vi "Trapezoidal Acceleration.vi"(9 "Desired":dbl, 10 "Actual":dbl) -> (2 "New Actual":dbl)   [LabVIEW 2013]
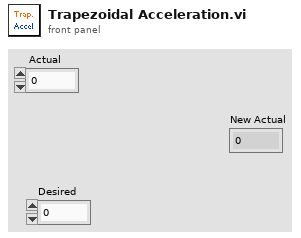
[diagram p1: front panel]
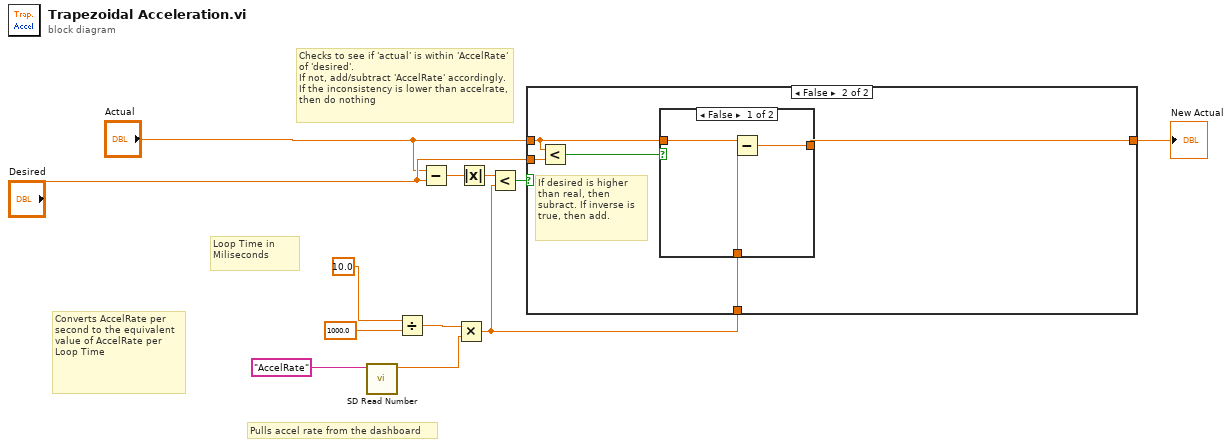
[diagram p0: block diagram]
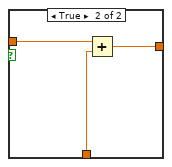
[diagram p3: hidden frame]
diagram:
  # "Pulls accel rate from the dashboard"
  # "Checks to see if 'actual' is within 'AccelRate' of 'desired'.\nIf not, add/subtract 'AccelRate' accordingly. If the inconsistency is lower than accelrate, then do nothing"
  # "Converts AccelRate per second to the equivalent value of AccelRate per Loop Time"
  # "Loop Time in Miliseconds"
  n1 = call <vilib>:"SD Read Number.vi"("Name"="AccelRate") -> ("Numeric"=w2:dbl)  [unwired: 8 in, 2 out]
  n2 = Divide(x=10.0, y=1000.0) -> (x/y=w8:dbl)
  n3 = Subtract(x="Actual", y="Desired") -> (x-y=w11:dbl)
  n4 = Multiply(x=w8, y=w2) -> (x*y=w6:dbl)
  n5 = Absolute Value(x=w11) -> (abs(x)=w12:dbl)
  n6 = Less?(x=w12, y=w6) -> (x < y?=w10:bool)
  n7 = case shown="False" w10 {
    tunnel: [w13 w18] -> w5
    tunnel: "Actual" -> [w13 w17]
    tunnel: "Desired" -> [_ w15]
    tunnel: w6 -> [_ w14]
    frame True {
    }
    frame False {
      # "If desired is higher than real, then subract. If inverse is true, then add."
      n8 = Less?(x=w17, y=w15) -> (x < y?=w16:bool)
      n9 = case shown="False" w16 {
        tunnel: w17 -> [w19 w23]
        tunnel: [w21 w24] -> w18
        tunnel: w14 -> [w20 w22]
        frame False {
          n10 = Subtract(x=w19, y=w20) -> (x-y=w21:dbl)
        }
        frame True {
          n11 = Add(x=w23, y=w22) -> (x+y=w24:dbl)
        }
      }
    }
  }
  "New Actual" <- w5
